vi "Get Assert Event Reference.vi"(7 "Action":T1, 8 "error in (no error)":errorcluster) -> (0 "error out":errorcluster, 3 "Assert Message Event":refnum<user-event>)   [LabVIEW 2016, in "Assert API Components.lvlib"]
uses:
  Assert API Components.lvlib
  Assert Event Actions.ctl
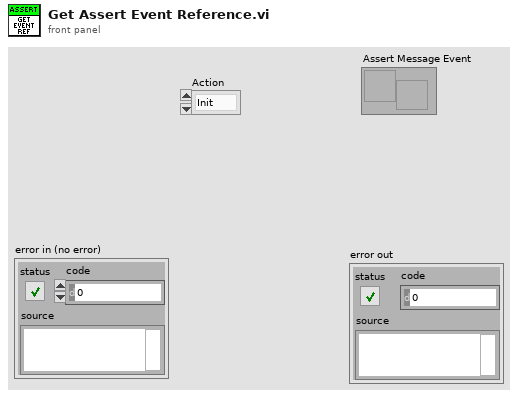
[diagram p1: front panel]
types:
  T1 = typedef "Assert API Components.lvlib/Assert Event Actions.ctl" = enum16{"Init", "Read", "Destroy"}
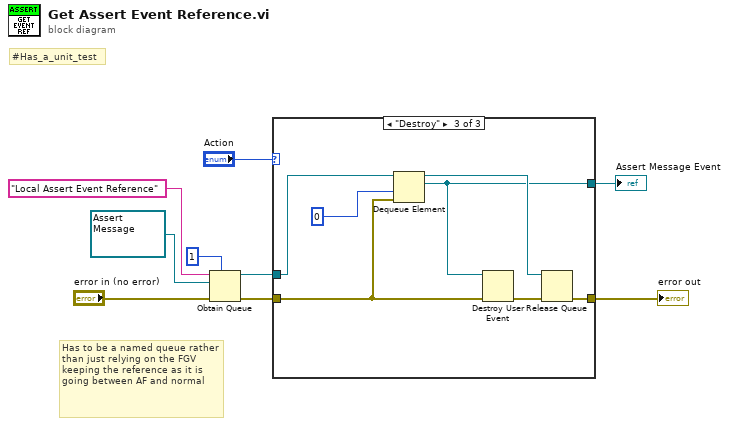
[diagram p0: block diagram]
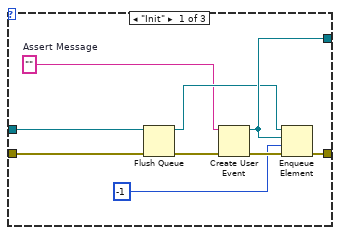
[diagram p2: hidden frame]
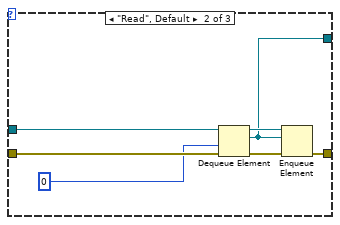
[diagram p3: hidden frame]
diagram:
  # "#Has_a_unit_test"
  # "Has to be a named queue rather than just relying on the FGV keeping the reference as it is going between AF and normal"
  n1 = Obtain Queue(max queue size (-1, unlimited)=1, name (unnamed)="Local Assert Event Reference", element data type=refnum<user-event> refnum ("Assert Message Event"), error in (no error)="error in (no error)") -> (queue out=w2:refnum<queue>, error out=w7:errorcluster)  [unwired: 1 in, 1 out]
  n2 = case shown="\"Destroy\"" "Action" {
    tunnel: [w17 w20 w30] -> w1
    tunnel: [w16 w19 w28] -> w9
    tunnel: w7 -> [w12 w24 w27]
    tunnel: w2 -> [w14 w25 w32]
    frame "Init" {
      w10 = ""  # Assert Message
      n3 = Flush Queue(queue=w14, error in (no error)=w12) -> (queue out=w13:refnum<queue>, error out=w11:errorcluster)  [unwired: 1 out]
      n4 = Create User Event(user event datatype=w10, error in=w11) -> (user event=w16:refnum<user-event>, error out=w18:errorcluster)
      n5 = Enqueue Element(queue=w13, element=w16, timeout in ms (-1)=-1, error in (no error)=w18) -> (error out=w17:errorcluster)  [unwired: 2 out]
    }
    frame "Read", Default {
      n6 = Dequeue Element(queue=w25, timeout in ms (-1)=0, error in (no error)=w24) -> (queue out=w23:refnum<queue>, element=w19:refnum<user-event>, error out=w22:errorcluster)  [unwired: 1 out]
      n7 = Enqueue Element(queue=w23, element=w19, error in (no error)=w22) -> (error out=w20:errorcluster)  [unwired: 1 in, 2 out]
    }
    frame "Destroy" {
      n8 = Dequeue Element(queue=w32, timeout in ms (-1)=0, error in (no error)=w27) -> (queue out=w29:refnum<queue>, element=w28:refnum<user-event>)  [unwired: 2 out]
      n9 = Destroy User Event(user event=w28, error in=w27) -> (error out=w31:errorcluster)
      n10 = Release Queue(queue=w29, error in (no error)=w31) -> (error out=w30:errorcluster)  [unwired: 1 in, 2 out]
    }
  }
  "Assert Message Event" <- w9
  "error out" <- w1
